vi "Vector to cartez.vi"(2 "Vector":dbl, 3 "Angle [deg]":dbl) -> (0 "Length":dbl, 1 "Height":dbl)   [LabVIEW 2013]
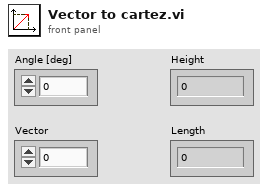
[diagram p1: front panel]
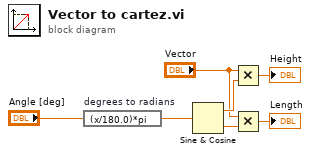
[diagram p0: block diagram]
diagram:
  n1 = expression code="(x/180.0)*pi" "degrees to radians"("Angle [deg]") -> (w7:dbl)
  n2 = Sine & Cosine(0:w7) -> (1:w6:dbl, 2:w5:dbl)
  n3 = Multiply(x="Vector", y=w6) -> (x*y=→"Height":dbl)
  n4 = Multiply(x="Vector", y=w5) -> (x*y=→"Length":dbl)
